vi "load_clz_data.vi"(7 "matched set":set{cluster{"CLZ id":i32, "CV id":i32}}(c389), 8 "error in (no error)":errorcluster, 10 "report path":path=path "D:/Comics/data/Complete_CLZ_collection.csv", 11 "Volumes in":refnum<class "CLZ Comics.lvclass">) -> (0 "error out":errorcluster, 3 "Volumes out":refnum<class "CLZ Comics.lvclass">)   [LabVIEW 2024, in "CLZ_to_ComicVine.lvlib" / "CLZ Comics.lvclass"]
uses:
  CLZ Comics.lvclass
  CLZ Comics.lvclass/CLZ Comics.ctl
  typedefs/volume--cluster.ctl
  typedefs/issue_number--cluster.ctl
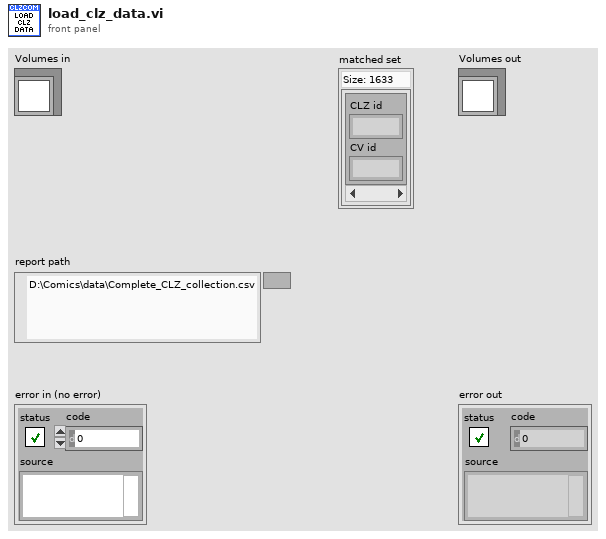
[diagram p1: front panel]
types:
  T1 = typedef "CLZ_to_ComicVine.lvlib/CLZ Comics.lvclass/issue_number--cluster.ctl" = cluster{"numeric":dbl, "issue":string, "variant":string}
  T2 = typedef "CLZ_to_ComicVine.lvlib/CLZ Comics.lvclass/volume--cluster.ctl" = cluster{"id":i32, "name":string, "issues":T1[], "matched":bool}
  T3 = typedef "CLZ_to_ComicVine.lvlib/CLZ_comic--cluster.ctl" = cluster{"Series":string, "Core SeriesID":i32, "Core ComicID":i32, "Issue":string, "Variant":string}
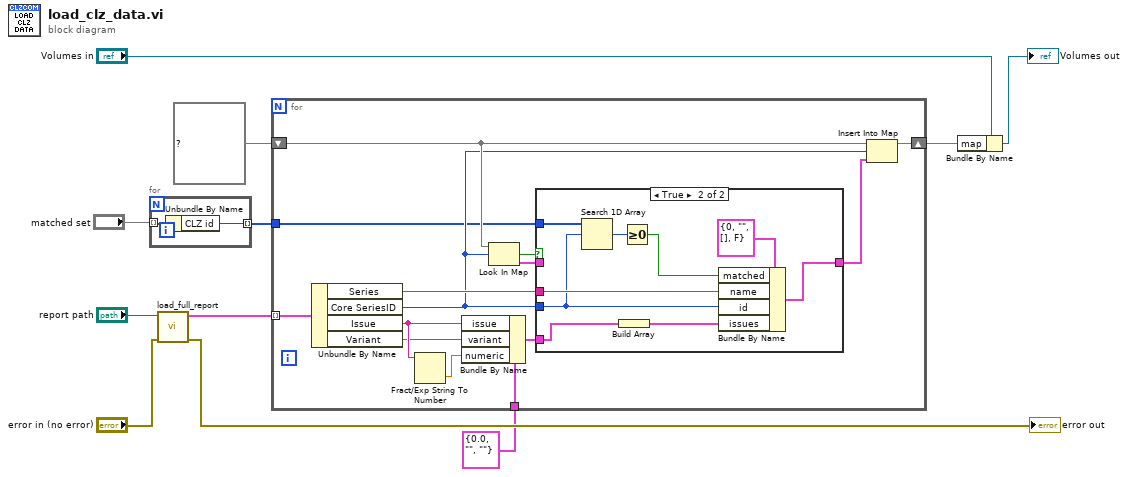
[diagram p0: block diagram]
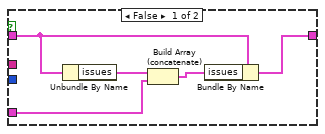
[diagram p2: hidden frame]
diagram:
  n1 = for {
    tunnel: "matched set" -> [w13] mode=indexing
    tunnel: [w12] -> w2 mode=indexing
    n2 = Unbundle By Name(w13) -> ("CLZ id"=w12:i32)
  }
  n3 = call "load_full_report.vi"("error in (no error)"="error in (no error)", "report path"="report path") -> ("error out"=→"error out":errorcluster, "clz_comics"=w8:T3[])  [unwired: 8 in]
  n4 = for {
    tunnel: w8 -> [w27] mode=indexing
    shift-right: [w21] -> w4
    shift-left: map{i32, T2} {} ("map") -> [w24]
    tunnel: w2 -> [w19]
    tunnel: T1 {"numeric"=0.0, "issue"="", "variant"=""} ("issue number") -> [w18]
    n5 = Unbundle By Name(w27) -> ("Series"=w25:string, "Core SeriesID"=w23:i32, "Issue"=w16:string, "Variant"=w15:string)
    n6 = Fract/Exp String To Number(string=w16) -> (number=w17:dbl)  [unwired: 3 in, 1 out]
    n7 = Bundle By Name(cluster=w18, "issue"=w16, "variant"=w15, "numeric"=w17) -> (w14:T1)
    n8 = Look In Map(map=w24, key=w23) -> (key not found?=w26:bool, value=w20:T2)  [unwired: 1 in]
    n9 = case shown="True" w26 {
      tunnel: w25 -> [_ w41]
      tunnel: w23 -> [_ w37]
      tunnel: [w31 w40] -> w22
      tunnel: w20 -> [w32 _]
      tunnel: w19 -> [_ w38]
      tunnel: w14 -> [w28 w34]
      frame False {
        n10 = Unbundle By Name(w32) -> ("issues"=w30:T1[])
        n11 = Build Array (concatenate)(w30, w28) -> (w29:T1[])
        n12 = Bundle By Name(cluster=w32, "issues"=w29) -> (w31:T2)
      }
      frame True {
        n13 = Search 1D Array(1D array=w38, element=w37) -> (index of element=w36:i32)  [unwired: 1 in]
        n14 = Build Array(w34) -> (w33:T1[])
        n15 = Greater Or Equal To 0?(x=w36) -> (x >= 0?=w35:bool)
        n16 = Bundle By Name(cluster=T2 {"id"=0, "name"="", "issues"=[], "matched"=FALSE} ("volume"), "matched"=w35, "name"=w41, "id"=w37, "issues"=w33) -> (w40:T2)
      }
    }
    n17 = Insert Into Map(map in=w24, key=w23, value=w22) -> (map out=w21:map{i32, T2})  [unwired: 2 out]
  }
  n18 = Bundle By Name(cluster="Volumes in", "map"=w4) -> (→"Volumes out":refnum<class "CLZ Comics.lvclass">)
